vi "Scan and Trace(Normal Draft).vi"() -> ()   [LabVIEW 2020]
uses:
  <vilib>/Utility/error.llb/DialogType.ctl
  Global Parameters.vi
  <vilib>/DAQmx/miscellaneous.llb/DAQmx Fill In Error Info.vi
  <vilib>/DAQmx/configure/timing.llb/DAQmx Timing (Sample Clock).vi
  <vilib>/DAQmx/read.llb/DAQmx Read (Counter 1D U32 1Chan NSamp).vi
  <vilib>/DAQmx/create/channels.llb/DAQmx Create Channel (CI-Count Edges).vi
  <vilib>/Utility/file.llb/Write Delimited Spreadsheet (DBL).vi
  <resource>/objmgr/daqmx.rc
panel:
  out "Read + Move Time":u32=103
  out "Laser On":bool
  out "Current Position":dbl[](array[numeric])=[100.0, 99.99645996, 110.0]
  in  "stop":bool
  in  "Tab Control":T1(tab)
  in  "Graph path":path=path "I:/scan map test"
  out "Intensity Graph":dbl[][](graph)=[[95300.0, 98850.0, 103700.0, 104550.0, 102500.0, 51500.0, 51850.0, 19000.0, 20650.0, 15000.0, 15300.0, 17150.0, 16250.0, 17200.0, 14950.0, 15050.0, 17650.0, 15350.0, 14300.0, 14550.0, 15700.0], [77600.0, 97750.0, 99400.0, 99250.0, 95500.0, 53250.0, 25650.0, 18800.0, 17350.0, 14250.0, 17250.0, 16050.0, 15600.0, 15200.0, 15250.0, 15700.0, 15150.0, 14650.0, 15600.0, 15700.0, 16550.0], [97000.0, 96100.0, 101550.0, 99100.0, 97250.0, 50150.0, 23650.0, 21050.0, 17550.0, 15950.0, 15300.0, 14700.0, 15200.0, 16950.0, 14500.0, 15450.0, 14550.0, 17050.0, 14550.0, 14900.0, 16600.0], [95600.0, 95800.0, 102500.0, 99350.0, 94900.0, 52700.0, 26600.0, 21250.0, 16250.0, 16150.0, 14800.0, 15550.0, 15800.0, 16350.0, 15400.0, 15850.0, 14500.0, 14750.0, 15550.0, 15750.0, 14900.0], [100050.0, 96100.0, 94400.0, 100500.0, 94450.0, 54350.0, 23850.0, 18950.0, 16100.0, 14850.0, 16700.0, 14950.0, 14250.0, 16700.0, 16100.0, 15700.0, 16450.0, 14650.0, 16950.0, 14000.0, 15800.0], [100300.0, 96050.0, 96850.0, 98000.0, 90700.0, 51250.0, 23450.0, 18050.0, 18300.0, 17300.0, 17050.0, 16300.0, 15950.0, 14850.0, 15500.0, 16450.0, 16200.0, 17200.0, 16450.0, 15300.0, 17100.0], [95650.0, 95650.0, 100700.0, 98700.0, 94500.0, 53950.0, 25250.0, 18850.0, 17150.0, 16050.0, 15050.0, 15450.0, 16050.0, 14600.0, 16500.0, 16350.0, 15500.0, 15450.0, 15300.0, 15150.0, 15650.0], [96700.0, 96200.0, 96650.0, 103650.0, 93400.0, 53300.0, 22500.0, 19050.0, 15850.0, 15350.0, 16550.0, 15200.0, 15250.0, 15400.0, 16550.0, 13950.0, 15150.0, 15600.0, 15150.0, 14500.0, 15900.0], [97500.0, 98050.0, 101500.0, 101650.0, 97000.0, 53700.0, 23400.0, 19450.0, 16700.0, 16850.0, 16450.0, 16250.0, 15900.0, 14600.0, 15700.0, 15400.0, 14900.0, 15950.0, 15450.0, 16050.0, 16100.0], [95400.0, 97550.0, 102050.0, 98600.0, 92100.0, 61200.0, 24550.0, 20500.0, 16000.0, 15350.0, 14450.0, 14150.0, 15750.0, 15950.0, 15750.0, 14800.0, 15000.0, 16150.0, 17250.0, 15350.0, 17400.0], [95750.0, 92950.0, 96100.0, 96550.0, 92550.0, 90100.0, 21900.0, 23000.0, 15000.0, 15550.0, 16000.0, 16000.0, 15400.0, 14150.0, 14350.0, 15950.0, 17250.0, 15750.0, 16100.0, 15300.0, 14400.0]]
  in  "go to crusor":bool caption="X"
  in  "vertical num":u32=20
  in  "horizontal num":u32=10
  out "horizontal range":dbl=50.0
  in  "horizontal start":dbl=50.0
  out "vertical range":dbl=200.0
  in  "vertical start":dbl
  in  "Horizontal axis":i8(ring) items=["x", "y", "z", ""]
  in  "Vertical axis":i8(ring)=2 items=["x", "y", "z", ""]
  out "vertical step":dbl=10.0
  out "horizontal step":dbl=5.0
  in  "Stop scan":bool
  out "counts/s":dbl=14400.0 format="%#.10g"
  out "H goal position":dbl[](array[numeric])=[50.0, 55.0, 60.0, 65.0, 70.0, 75.0, 80.0, 85.0, 90.0, 95.0, 100.0]
  out "V goal position":dbl[](array[numeric])=[0.0, 10.0, 20.0, 30.0, 40.0, 50.0, 60.0, 70.0, 80.0, 90.0, 100.0, 110.0, 120.0, 130.0, 140.0, 150.0, 160.0, 170.0, 180.0, 190.0, 200.0]
  out "Loop  indicator":i32=2147483647
  in  "horizontal end":dbl=50.0
  in  "vertical end":dbl=200.0
  out "Waveform Chart":dbl(graph)=93500.0
  in  "Start moving":bool=TRUE
  in  "Save trace data?":bool
  in  "-0.05 2":bool caption="X"
  in  "Tracing axis":enum16{"x", "y", "z"}(ring)=enum."z"
  in  "-01 2":bool caption="X"
  in  "Wait time(ms)":u32
  in  "+01 2":bool caption="X"
  in  "+0.05 2":bool caption="X"
  in  "-0.01 2":bool caption="X"
  in  "+0.01 2":bool caption="X"
  in  "Exit Tracing":bool
  out "counts rate":dbl=93500.0 format="%#.10g"
  in  "Trace data file path 2":path=path "trace data"
  in  "set trace data save rate(ms)":u32
  in  "Stop Counts":bool
  out "Actual Duty Cycle":dbl=0.5
  out "Actual Frequency":dbl=50.0
  out "Duty Cycle":dbl=0.5 format="%.6f"
  out "Frequency":dbl=50.0 format="%.6f"
  out "Output Terminal":tag="/Dev1/PFI2"
  out "Counter":tag="Dev1/ctr0"
  out "Clock on":bool
  out "ASG连接状态":bool
  out "ASG error":errorcluster
  out "Scanner\n error":errorcluster
  out "Sample Clock Source":tag="/Dev1/PFI2"
  out "Sample Rate":dbl=50.0
  in  "Counter 2":tag="Dev1/ctr1"
  in  "Input Terminal":tag="/Dev1/PFI12"
  in  "Samples":i32=2
  out "Data":u32[](array[numeric])=[293, 581]
  in  "Active Edge":i32(ring)=10280 items=["Rising"=10280, "Falling"=10171]
  in  "Sample Mode":i32(ring)=10178 items=["Finite Samples"=10178, "Continuous Samples"=10123, "Hardware Timed Single Point"=12522]
  in  "milliseconds to wait":u32
  out "Position After move":dbl[](array[numeric]) format="%.6f"
  out "Position After move 2":dbl[](array[numeric]) format="%.6f"
  in  "start":bool
  in  "Select Process Before Start":enum16{"Goto cursor", "Trace", "Scan"}(ring)=enum."Trace"
  out "Scanning":bool
  out "Tracing":bool
  out "Goto cursor":bool
  # "Only for showing Clock Settings, Please go to Global Parameter to Change the Settings"
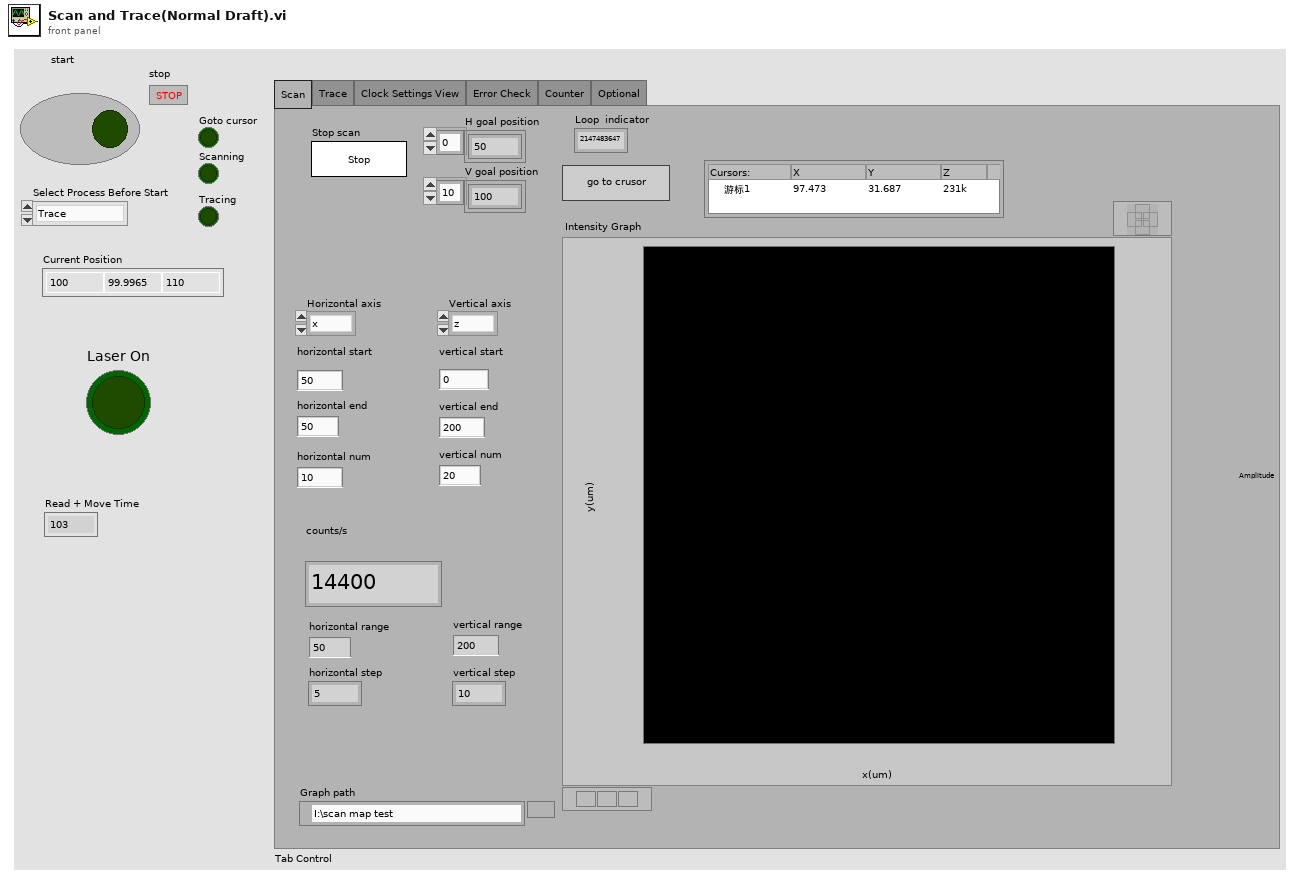
[diagram p1: front panel]
types:
  T1 = enum32{"Scan", "Trace", "Clock Settings View", "Error Check", "Counter", "Optional"}
  T2 = typedef "DialogType.ctl" = u16
  T3 = typedef "imagedata.ctl" = cluster{"image type":i32, "image depth":i32, "image":u8[], "mask":u8[], "colors":u32[], "Rectangle":cluster{"left":i16, "top":i16, "right":i16, "bottom":i16}}
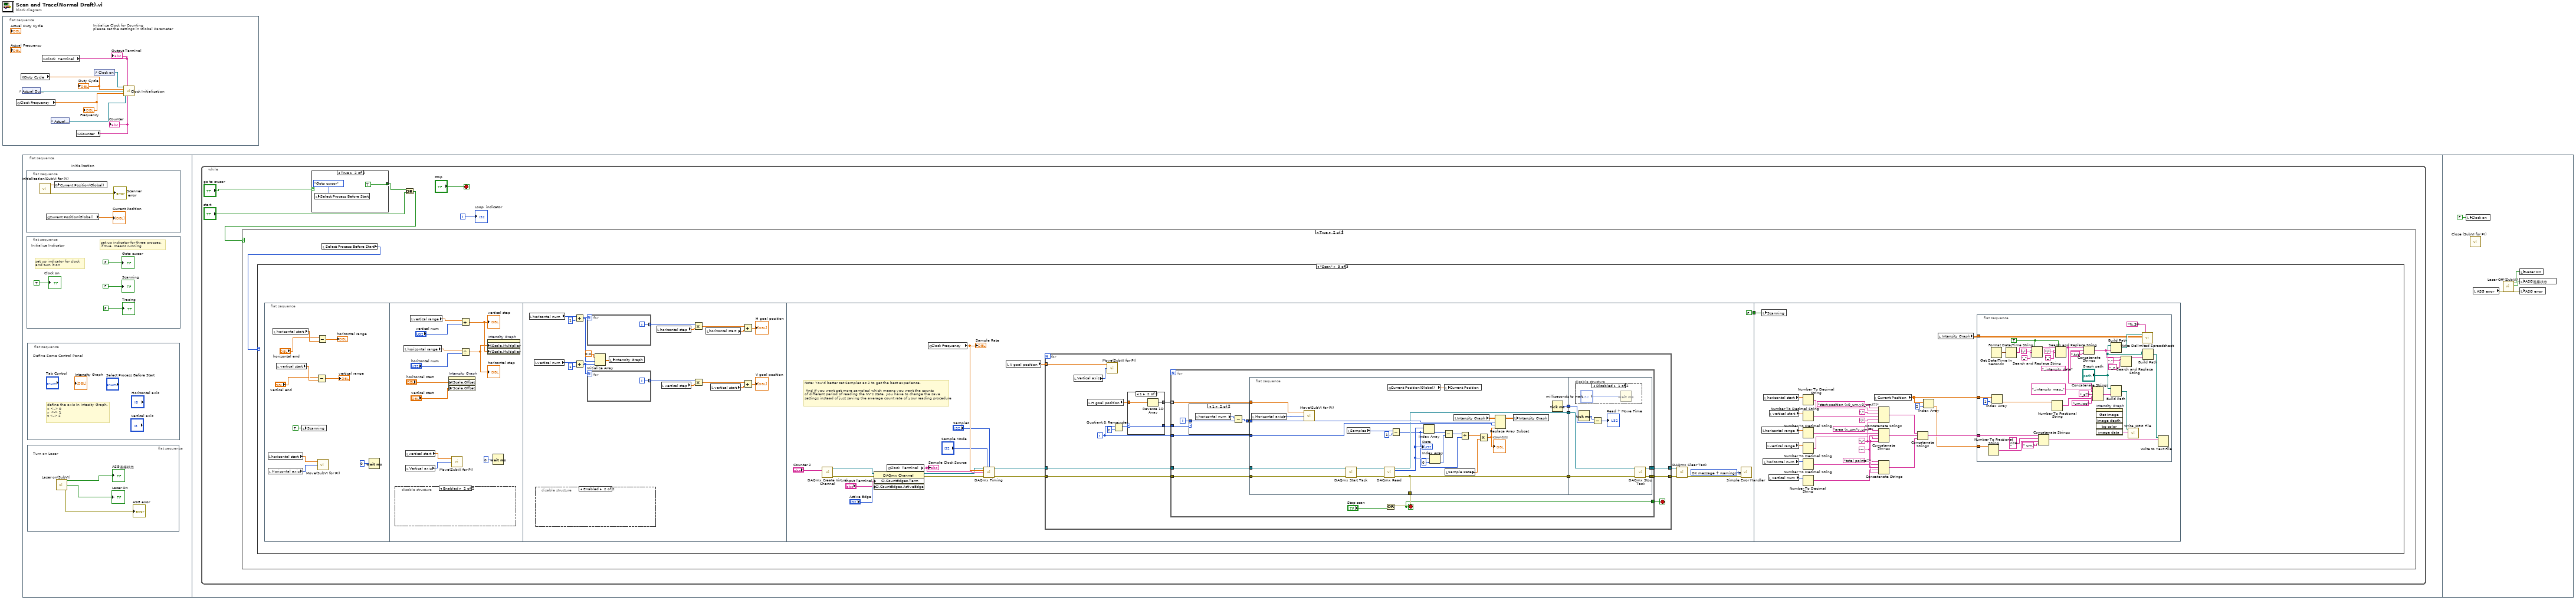
[diagram p0: block diagram]
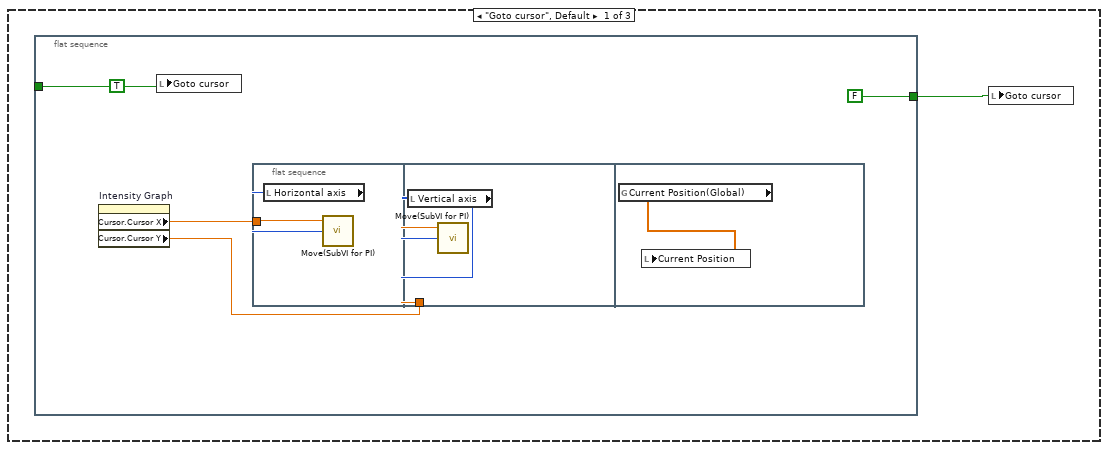
[diagram p3: hidden frame]
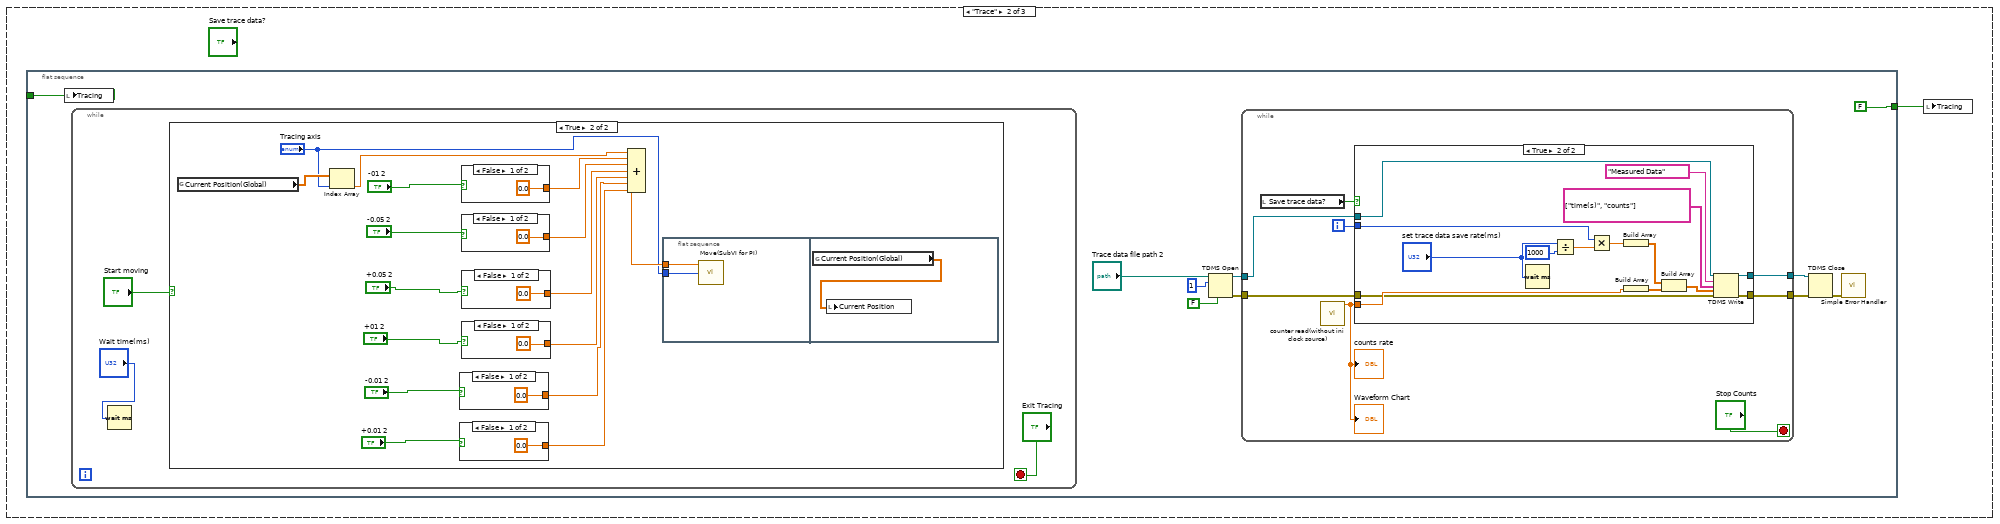
[diagram p4: hidden frame]
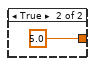
[diagram p7: hidden frame]
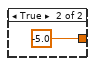
[diagram p8: hidden frame]
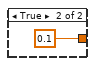
[diagram p9: hidden frame]
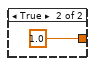
[diagram p10: hidden frame]
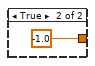
[diagram p11: hidden frame]
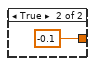
[diagram p12: hidden frame]
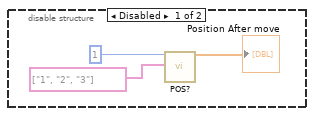
[diagram p13: hidden frame]
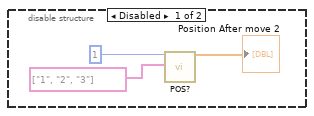
[diagram p14: hidden frame]
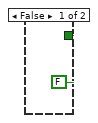
[diagram p18: hidden frame]
diagram:
  n1 = flat-sequence {
    frame #0 {
      # "Initialize Clock for Counting\nplease set the settings in Global Parameter"
      n2 = global read "Global Parameters.vi" "Clock Frequency"() -> (w3:dbl)
      "Frequency" <- w3
      n3 = global read "Global Parameters.vi" "Duty Cycle"() -> (w4:dbl)
      "Duty Cycle" <- w4
      n4 = control-ref of="Actual Duty Cycle"() -> (w1:refnum<vi>)
      n5 = global read "Global Parameters.vi" "Clock  Terminal"() -> (w5:tag)
      "Output Terminal" <- w5
      n6 = control-ref of="Actual Frequency"() -> (w2:refnum<vi>)
      n7 = global read "Global Parameters.vi" "Counter"() -> (w6:tag)
      "Counter" <- w6
      n8 = control-ref of="Clock on"() -> (w7:refnum<vi>)
      n9 = call "Clock Initialization.vi"("Boolean in"=w7, "Output Terminal"=w5, "Duty Cycle"=w4, "Actual Duty Cycle"=w1, "Frequency"=w3, "Actual Frequency"=w2, "Counter"=w6) -> ()  [unwired: 9 in]
    }
  }
  n10 = flat-sequence {
    frame #0 {
      # "Initialization"
      n11 = flat-sequence {
        frame #0 {
          n12 = call "Initialization(SubVI for PI).vi"() -> ("error out"=→"Scanner\n error":errorcluster, "Position"=w16:dbl[])  [unwired: 10 in]
          n13 = global read "Global Parameters.vi" "Current Position(Global)"() -> (→"Current Position":dbl[])
          n14 = global write "Global Parameters.vi" "Current Position(Global)"(w16) -> ()
        }
      }
      n15 = flat-sequence {
        frame #0 {
          # "Initialize Indicator"
          # "set up indicator for clock \nand turn it on"
          # "set up indicator for three prosses,\nif true, means running"
          "Goto cursor" <- FALSE
          "Tracing" <- FALSE
          "Scanning" <- FALSE
          "Clock on" <- TRUE
        }
      }
      n16 = flat-sequence {
        frame #0 {
          # "Define Some Control Panel"
          # "define the axis in Intesity Graph,\nx <-> 0\ny <-> 1\nz <-> 2"
        }
      }
      n17 = flat-sequence {
        frame #0 {
          # "Turn on Laser"
          n18 = call "Laser on(SubVI).vi"() -> ("error out"=→"ASG error":errorcluster, "Laser On"=→"Laser On":bool, "ASG Connection On?"=→"ASG连接状态":bool)  [unwired: 9 in]
        }
      }
    }
    frame #1 {
      n19 = while {
        i -> [w21]
        stop <- "stop" stop-if-true
        n20 = case shown="True" "go to crusor" {
          tunnel: [FALSE TRUE] -> w19
          frame False {
          }
          frame True {
            n21 = local write "Select Process Before Start"(enum16{"Goto cursor", "Trace", "Scan"}."Goto cursor" ("Select Process Before Start")) -> ()
          }
        }
        n22 = Or(x=w19, y="start") -> (x .or. y?=w18:bool)
        n23 = case shown="True" w18 {
          frame False {
          }
          frame True {
            n24 = local read "Select Process Before Start"() -> (w24:enum16{"Goto cursor", "Trace", "Scan"})
            n25 = case shown="\"Scan\"" w24 {
              frame "Goto cursor", Default {
                n26 = flat-sequence {
                  tunnel: TRUE -> [w28]
                  tunnel: [FALSE] -> w25
                  frame #0 {
                    n27 = property on="Intensity Graph" class="IntGraph (strict)"() -> ("Cursor.Cursor X"=w30:dbl, "Cursor.Cursor Y"=w29:dbl)  [unwired: 2 in, 2 out]
                    n28 = local write "Goto cursor"(w28) -> ()
                    n29 = flat-sequence {
                      tunnel: w30 -> [w32]
                      tunnel: w29 -> [w34]
                      frame #0 {
                        n30 = local read "Horizontal axis"() -> (w31:i8)
                        n31 = call "Move(SubVI for PI).vi"("Goal"=w32, "index"=w31) -> ()  [unwired: 5 in, 1 out]
                      }
                      frame #1 {
                        n32 = local read "Vertical axis"() -> (w33:i8)
                        n33 = call "Move(SubVI for PI).vi"("Goal"=w34, "index"=w33) -> ()  [unwired: 5 in, 1 out]
                      }
                      frame #2 {
                        n34 = global read "Global Parameters.vi" "Current Position(Global)"() -> (w35:dbl[])
                        n35 = local write "Current Position"(w35) -> ()
                      }
                    }
                  }
                }
                n36 = local write "Goto cursor"(w25) -> ()
              }
              frame "Trace" {
                n37 = flat-sequence {
                  tunnel: [FALSE] -> w37
                  tunnel: TRUE -> [w38]
                  frame #0 {
                    n38 = local write "Tracing"(w38) -> ()
                    n39 = while {
                      stop <- "Exit Tracing" stop-if-true
                      n40 = Wait (ms)(milliseconds to wait="Wait time(ms)") -> ()  [unwired: 1 out]
                      n41 = case shown="True" "Start moving" {
                        frame False {
                        }
                        frame True {
                          n42 = global read "Global Parameters.vi" "Current Position(Global)"() -> (w91:dbl[])
                          n43 = Index Array(array=w91, index="Tracing axis") -> (element=w84:dbl)
                          n44 = case shown="False" "-0.01 2" {
                            tunnel: [0.0 -5.0] -> w86
                            frame False {
                            }
                            frame True {
                            }
                          }
                          n45 = case shown="False" "+0.01 2" {
                            tunnel: [0.0 5.0] -> w85
                            frame False {
                            }
                            frame True {
                            }
                          }
                          n46 = case shown="False" "-01 2" {
                            tunnel: [0.0 -0.1] -> w90
                            frame False {
                            }
                            frame True {
                            }
                          }
                          n47 = case shown="False" "-0.05 2" {
                            tunnel: [0.0 -1.0] -> w89
                            frame False {
                            }
                            frame True {
                            }
                          }
                          n48 = case shown="False" "+0.05 2" {
                            tunnel: [0.0 1.0] -> w88
                            frame False {
                            }
                            frame True {
                            }
                          }
                          n49 = case shown="False" "+01 2" {
                            tunnel: [0.0 0.1] -> w87
                            frame False {
                            }
                            frame True {
                            }
                          }
                          n50 = Compound Arithmetic op=ADD(w84, w90, w89, w88, w87, w86, w85) -> (w77:dbl)
                          n51 = flat-sequence {
                            tunnel: w77 -> [w105]
                            tunnel: "Tracing axis" -> [w104]
                            frame #0 {
                              n52 = call "Move(SubVI for PI).vi"("Goal"=w105, "index"=w104) -> ()  [unwired: 5 in, 1 out]
                            }
                            frame #1 {
                              n53 = global read "Global Parameters.vi" "Current Position(Global)"() -> (w106:dbl[])
                              n54 = local write "Current Position"(w106) -> ()
                            }
                          }
                        }
                      }
                    }
                    n55 = TDMS Open(6:FALSE ("disable buffering (T)"), 10:1, 11:"Trace data file path 2") -> (0:w45:errorcluster, 3:w44:refnum<k34>)  [unwired: 4 in]
                    n56 = while {
                      tunnel: w45 -> [w54]
                      tunnel: w44 -> [w53]
                      tunnel: [w50] -> w42
                      tunnel: [w49] -> w41
                      i -> [w55]
                      stop <- "Stop Counts" stop-if-true
                      n57 = local read "Save trace data?"() -> (w51:bool)
                      n58 = call "counter read(without ini clock source).vi"() -> ("counter rate"=w52:dbl)  [unwired: 11 in]
                      "counts rate" <- w52
                      "Waveform Chart" <- w52
                      n59 = case shown="True" w51 {
                        tunnel: w53 -> [w57 w64]
                        tunnel: [w57 w63] -> w50
                        tunnel: w52 -> [_ w62]
                        tunnel: w54 -> [w56 w61]
                        tunnel: [w56 w60] -> w49
                        tunnel: w55 -> [_ w59]
                        frame False {
                        }
                        frame True {
                          n60 = Wait (ms)(milliseconds to wait="set trace data save rate(ms)") -> ()  [unwired: 1 out]
                          n61 = Divide(x="set trace data save rate(ms)", y=u32 1000) -> (x/y=w66:dbl)
                          n62 = Multiply(x=w59, y=w66) -> (x*y=w65:dbl)
                          n63 = Build Array(w65) -> (w70:dbl[])
                          n64 = Build Array(w62) -> (w69:dbl[])
                          n65 = Build Array(w70, w69) -> (w68:dbl[][])
                          n66 = TDMS Write(0:w64, 5:"Measured Data" ("group name"), 7:string[] ["time(s)", "counts"] ("channel names"), 9:w68, 11:w61) -> (4:w63:refnum<k34>, 15:w60:errorcluster)  [unwired: 1 in, 2 out]
                        }
                      }
                    }
                    n67 = TDMS Close(8:w41, 11:w42) -> (0:w43:errorcluster)  [unwired: 1 out]
                    n68 = call <vilib>:"Simple Error Handler.vi"("error in (no error)"=w43) -> ()  [unwired: 1 in, 8 out]
                  }
                }
                n69 = local write "Tracing"(w37) -> ()
              }
              frame "Scan" {
                n70 = flat-sequence {
                  tunnel: [FALSE] -> w107
                  tunnel: w107 -> [w271]
                  frame #0 {
                    n71 = local read "horizontal start"() -> (w109:dbl)
                    n72 = local read "Horizontal axis"() -> (w110:i8)
                    n73 = local read "horizontal start"() -> (w114:dbl)
                    n74 = local read "vertical start"() -> (w112:dbl)
                    n75 = local write "Scanning"(TRUE) -> ()
                    n76 = Subtract(x="vertical end", y=w112) -> (x-y=→"vertical range":dbl)
                    n77 = Subtract(x="horizontal end", y=w114) -> (x-y=→"horizontal range":dbl)
                    n78 = call "Move(SubVI for PI).vi"("Goal"=w109, "index"=w110) -> ()  [unwired: 5 in, 1 out]
                    n79 = Wait (ms)(milliseconds to wait=u32 0 ("milliseconds to wait 2")) -> ()  [unwired: 1 out]
                  }
                  frame #1 {
                    n80 = disable-structure shown="Enabled" {
                      frame Disabled {
                        n81 = call "POS?.vi"("System no."=1, "Axes to query"=string[] ["1", "2", "3"] ("String")) -> ("Position"=→"Position After move":dbl[])  [unwired: 3 in, 14 out]
                      }
                      frame Enabled {
                      }
                    }
                    n82 = local read "horizontal range"() -> (w122:dbl)
                    n83 = local read "vertical start"() -> (w119:dbl)
                    n84 = local read "Vertical axis"() -> (w120:i8)
                    n85 = local read "vertical range"() -> (w121:dbl)
                    n86 = property on="Intensity Graph" class="IntGraph (strict)"("XScale.Offset"="horizontal start", "YScale.Offset"="vertical start") -> ()  [unwired: 2 in, 2 out]
                    n87 = call "Move(SubVI for PI).vi"("Goal"=w119, "index"=w120) -> ()  [unwired: 5 in, 1 out]
                    n88 = Divide(x=w121, y="vertical num") -> (x/y=w123:dbl)
                    "vertical step" <- w123
                    n89 = Divide(x=w122, y="horizontal num") -> (x/y=w124:dbl)
                    "horizontal step" <- w124
                    n90 = property on="Intensity Graph" class="IntGraph (strict)"("XScale.Multiplier"=w124, "YScale.Multiplier"=w123) -> ()  [unwired: 2 in, 2 out]
                    n91 = Wait (ms)(milliseconds to wait=u32 0 ("milliseconds to wait 2")) -> ()  [unwired: 1 out]
                  }
                  frame #2 {
                    n92 = local read "horizontal num"() -> (w134:u32)
                    n93 = local read "vertical num"() -> (w137:u32)
                    n94 = disable-structure shown="Enabled" {
                      frame Disabled {
                        n95 = call "POS?.vi"("System no."=1, "Axes to query"=string[] ["1", "2", "3"] ("String")) -> ("Position"=→"Position After move 2":dbl[])  [unwired: 3 in, 14 out]
                      }
                      frame Enabled {
                      }
                    }
                    n96 = Add(x=w134, y=1) -> (x+y=w133:u32)
                    n97 = Add(x=w137, y=1) -> (x+y=w132:u32)
                    n98 = for {
                      N: w133 -> [_]
                      tunnel: [w154] -> w149 mode=indexing
                      i -> [w154]
                    }
                    n99 = for {
                      N: w132 -> [_]
                      tunnel: [w153] -> w144 mode=indexing
                      i -> [w153]
                    }
                    n100 = Initialize Array(0.0, w133, w132) -> (w138:dbl[][])
                    n101 = local write "Intensity Graph"(w138) -> ()
                    n102 = local read "horizontal step"() -> (w148:dbl)
                    n103 = local read "vertical step"() -> (w143:dbl)
                    n104 = Multiply(x=w149, y=w148) -> (x*y=w147:dbl[])
                    n105 = Multiply(x=w144, y=w143) -> (x*y=w142:dbl[])
                    n106 = local read "horizontal start"() -> (w146:dbl)
                    n107 = local read "vertical start"() -> (w141:dbl)
                    n108 = Add(x=w147, y=w146) -> (x+y=→"H goal position":dbl[])
                    n109 = Add(x=w142, y=w141) -> (x+y=→"V goal position":dbl[])
                  }
                  frame #3 {
                    w170 = T2 3 items=["no dialog", "OK message", "continue or stop message", "OK message + warnings", "continue/stop + warnings"] ("type of dialog (OK msg:1)")
                    # "Note: You'd better set Samples as 2 to get the best experience,\n\n And if you want get more samples( which means you want the counts \nof different period of reading the NV's state, you have to change the save \nsettings instead of just saving the average count rate of your reading procedure"
                    n110 = call-poly <vilib>:"DAQmx Create Virtual Channel.vi"("counter"="Counter 2") -> ("task out"=w166:refnum<k21>, "error out"=w165:errorcluster)  [unwired: 13 in]
                    n111 = property class="DAQmx Channel"(reference=w166, error in=w165, "CI.CountEdges.Term"="Input Terminal", "CI.CountEdges.ActiveEdge"="Active Edge") -> (reference out=w158:refnum<k21>, error out=w157:errorcluster)
                    n112 = global read "Global Parameters.vi" "Clock  Terminal"() -> (w163:tag)
                    "Sample Clock Source" <- w163
                    n113 = global read "Global Parameters.vi" "Clock Frequency"() -> (w164:dbl)
                    "Sample Rate" <- w164
                    n114 = call-poly <vilib>:"DAQmx Timing.vi"("task/channels in"=w158, "sample mode"="Sample Mode", "samples per channel"="Samples", "rate"=w164, "source"=w163, "error in"=w157) -> ("task out"=w156:refnum<k21>, "error out"=w155:errorcluster)  [unwired: 8 in]
                    n115 = local read "V goal position"() -> (w173:dbl[])
                    n116 = for {
                      tunnel: w173 -> [w180] mode=indexing
                      tunnel: [w175] -> w162
                      tunnel: [w174] -> w161
                      tunnel: w156 -> [w177]
                      tunnel: w155 -> [w176]
                      i -> [w181]
                      stop <- w178 stop-if-true
                      n117 = local read "Vertical axis"() -> (w179:i8)
                      n118 = local read "H goal position"() -> (w185:dbl[])
                      n119 = call "Move(SubVI for PI).vi"("Goal"=w180, "index"=w179) -> ()  [unwired: 5 in, 1 out]
                      n120 = Quotient & Remainder(x=w181, y=2) -> (x-y*floor(x/y)=w184:i32)  [unwired: 1 out]
                      n121 = case shown="1" w184 {
                        selector: w184 -> [w239 w241]
                        tunnel: w185 -> [w240 w243]
                        tunnel: [w240 w242] -> w183
                        tunnel: [w239 w241] -> w182
                        frame 0, Default {
                        }
                        frame 1 {
                          n122 = Reverse 1D Array(array=w243) -> (reversed array=w242:dbl[])
                        }
                      }
                      n123 = for {
                        tunnel: w183 -> [w201] mode=indexing
                        tunnel: w182 -> [w200]
                        tunnel: w181 -> [w197]
                        tunnel: [w194] -> w178
                        tunnel: w177 -> [w193]
                        tunnel: w176 -> [w192]
                        tunnel: [w189] -> w175
                        tunnel: [w188] -> w174
                        i -> [w199]
                        stop <- w194 stop-if-true
                        n124 = case shown="1" w200 {
                          tunnel: w199 -> [w202 w204]
                          tunnel: [w202 w203] -> w198
                          frame 0, Default {
                          }
                          frame 1 {
                            n125 = local read "horizontal num"() -> (w205:u32)
                            n126 = Subtract(x=w205, y=w204) -> (x-y=w203:u32)
                          }
                        }
                        n127 = flat-sequence {
                          tunnel: [w221] -> w196
                          tunnel: [w222] -> w191
                          tunnel: [w221] -> w190
                          tunnel: [w208] -> w187
                          tunnel: w198 -> [w229]
                          tunnel: w201 -> [w207]
                          tunnel: w197 -> [w228]
                          tunnel: w193 -> [w224]
                          tunnel: w192 -> [w223]
                          tunnel: w191 -> [w236]
                          tunnel: w190 -> [w235]
                          tunnel: [w234] -> w189
                          tunnel: [w233] -> w188
                          tunnel: w187 -> [w232]
                          frame #0 {
                            n128 = local read "Horizontal axis"() -> (w206:i8)
                            n129 = call "Move(SubVI for PI).vi"("Goal"=w207, "index"=w206) -> ()  [unwired: 5 in, 1 out]
                            n130 = call <vilib>:"DAQmx Start Task.vi"("task/channels in"=w224, "error in"=w223) -> ("task out"=w210:refnum<k21>, "error out"=w209:errorcluster)  [unwired: 12 in]
                            n131 = local read "Samples"() -> (w215:i32)
                            n132 = call-poly <vilib>:"DAQmx Read.vi"("task/channels in"=w210, "error in"=w209) -> ("task out"=w222:refnum<k21>, "data"=w214:u32[], "error out"=w221:errorcluster)  [unwired: 11 in]
                            "Data" <- w214
                            n133 = global read "Global Parameters.vi" "Current Position(Global)"() -> (w226:dbl[])
                            n134 = Subtract(x=w215, y=1) -> (x-y=w211:i32)
                            n135 = Index Array(array=w214, index=w211) -> (element=w217:u32)
                            n136 = Index Array(array=w214, index=0) -> (element=w218:u32)
                            n137 = Subtract(x=w217, y=w218) -> (x-y=w216:u32)
                            n138 = local write "Current Position"(w226) -> ()
                            n139 = local read "Sample Rate"() -> (w212:dbl)
                            n140 = local read "Intensity Graph"() -> (w230:dbl[][])
                            n141 = Divide(x=w216, y=w211) -> (x/y=w213:dbl)
                            n142 = Multiply(x=w213, y=w212) -> (x*y=w225:dbl)
                            "counts/s" <- w225
                            n143 = Replace Array Subset(array=w230, new element=w225, index (row)=w229, index (col)=w228) -> (w227:dbl[][])
                            n144 = local write "Intensity Graph"(w227) -> ()
                            n145 = Tick Count (ms)() -> (millisecond timer value=w208:u32)
                          }
                          frame #1 {
                            n146 = disable-structure shown="Disabled" {
                              frame Disabled {
                                n147 = Wait (ms)(milliseconds to wait="milliseconds to wait") -> ()  [unwired: 1 out]
                              }
                              frame Enabled {
                              }
                            }
                            n148 = Tick Count (ms)() -> (millisecond timer value=w231:u32)
                            n149 = Subtract(x=w231, y=w232) -> (x-y=→"Read + Move Time":u32)
                            n150 = call <vilib>:"DAQmx Stop Task.vi"("task/channels in"=w236, "error in"=w235) -> ("task out"=w234:refnum<k21>, "error out"=w233:errorcluster)  [unwired: 12 in]
                          }
                        }
                        n151 = Or(x=w196, y="Stop scan") -> (x .or. y?=w194:bool)
                      }
                    }
                    n152 = call <vilib>:"DAQmx Clear Task.vi"("task in"=w162, "error in"=w161) -> ("error out"=w171:errorcluster)  [unwired: 13 in]
                    n153 = call <vilib>:"Simple Error Handler.vi"("type of dialog (OK msg:1)"=w170, "error in (no error)"=w171) -> ()  [unwired: 3 in, 5 out]
                  }
                  frame #4 {
                    w260 = "\r"
                    w262 = "*" ("string")
                    n154 = local write "Scanning"(w271) -> ()
                    n155 = local read "horizontal range"() -> (w249:dbl)
                    n156 = local read "horizontal num"() -> (w255:u32)
                    n157 = local read "horizontal start"() -> (w252:dbl)
                    n158 = local read "vertical range"() -> (w248:dbl)
                    n159 = local read "vertical num"() -> (w254:u32)
                    n160 = local read "vertical start"() -> (w251:dbl)
                    n161 = Number To Decimal String(number=w252) -> (decimal integer string=w269:string)  [unwired: 1 out]
                    n162 = Number To Decimal String(number=w251) -> (decimal integer string=w267:string)  [unwired: 1 out]
                    n163 = Number To Decimal String(number=w249) -> (decimal integer string=w264:string)  [unwired: 1 out]
                    n164 = Number To Decimal String(number=w248) -> (decimal integer string=w250:string)  [unwired: 1 out]
                    n165 = Number To Decimal String(number=w255) -> (decimal integer string=w261:string)  [unwired: 1 out]
                    n166 = Number To Decimal String(number=w254) -> (decimal integer string=w253:string)  [unwired: 1 out]
                    n167 = local read "Current Position"() -> (w244:dbl[])
                    n168 = Concatenate Strings("start position (x0_um,y0_um)=(" ("string"), w269, "," ("string"), w267, ")" ("string"), w260) -> (w259:string)
                    n169 = Concatenate Strings("area (x_um*y_um)=" ("string"), w264, w262, w250, w260) -> (w258:string)
                    n170 = Concatenate Strings("total points=" ("string"), w261, w262, w253, w260) -> (w257:string)
                    n171 = Concatenate Strings(w259, w258, w257) -> (w256:string)
                    n172 = Index Array(array=w244, index=2) -> (element=w246:dbl)
                    n173 = local read "Intensity Graph"() -> (w245:dbl[][])
                    n174 = flat-sequence {
                      tunnel: w245 -> [w274]
                      tunnel: w256 -> [w287]
                      tunnel: w246 -> [w285]
                      tunnel: w244 -> [w280]
                      frame #0 {
                        w277 = TRUE ("replace all? (F)")
                        n175 = Number To Fractional String(number=w285) -> (F-format string=w284:string)  [unwired: 3 in]
                        n176 = Get Date/Time In Seconds() -> (seconds since 1Jan1904=w307:timestamp)
                        n177 = Index Array(array=w280, index=2 ("索引")) -> (element=w278:dbl)
                        n178 = Format Date/Time String(seconds (now)=w307) -> (date/time string=w301:string)  [unwired: 2 out]
                        n179 = Search and Replace String(replace all?=w277, input string=w301, search string=":", replace string="_" ("replace string (\"\")")) -> (result string=w304:string)  [unwired: 1 in, 6 out]
                        n180 = Concatenate Strings(w287, "\nz=" ("字符串"), w284, " um." ("字符串")) -> (w286:string)
                        n181 = Number To Fractional String(number=w278) -> (F-format string=w281:string)  [unwired: 3 in]
                        n182 = Search and Replace String(replace all?=w277, input string=w304, search string="/", replace string="_" ("replace string (\"\")")) -> (result string=w292:string)  [unwired: 1 in, 6 out]
                        n183 = Concatenate Strings(w292, "_intensity date" ("string"), ".txt" ("string")) -> (w297:string)
                        n184 = Concatenate Strings(w292, "_intensity map_" ("string"), "_z=" ("字符串"), w281, "um.jpg" ("string")) -> (w300:string)
                        n185 = invoke on="Intensity Graph" class="IntGraph (strict)" method="Get Image"() -> ("image data"=w273:T3)  [unwired: 6 in, 5 out]
                        n186 = Build Path(base path="Graph path", name or relative path=w297) -> (appended path=w275:path)
                        n187 = Build Path(base path="Graph path", name or relative path=w300) -> (appended path=w299:path)
                        n188 = Search and Replace String(input string=w297, search string="." ("substring (\"\")"), replace string="_2." ("replace string (\"\")")) -> (result string=w294:string)  [unwired: 1 in, 7 out]
                        n189 = call <vilib>:"Write JPEG File.vi"("image data"=w273, "path to JPEG file"=w299) -> ()  [unwired: 1 in, 9 out]
                        n190 = call-poly <vilib>:"Write Delimited Spreadsheet.vi"("file path (dialog if empty)"=w275, "format (%.3f)"="%.3f", "2D data"=w274) -> ()  [unwired: 11 in, 2 out]
                        n191 = Build Path(base path="Graph path", name or relative path=w294) -> (appended path=w293:path)
                        n192 = Write to Text File(file (use dialog)=w293, text=w286) -> ()  [unwired: 1 in, 4 out]
                      }
                    }
                  }
                }
              }
            }
          }
        }
        "Loop  indicator" <- w21
      }
    }
    frame #2 {
      n193 = local write "Clock on"(FALSE) -> ()
      n194 = call "Close (SubVI for PI).vi"() -> ()  [unwired: 12 in]
      n195 = local read "ASG error"() -> (w311:errorcluster)
      n196 = call "Laser Off (SubVI).vi"("error in (no error)"=w311) -> ("error out"=w312:errorcluster, "ASG Connection on"=w313:bool, "Laser On"=w314:bool)  [unwired: 8 in]
      n197 = local write "Laser On"(w314) -> ()
      n198 = local write "ASG连接状态"(w313) -> ()
      n199 = local write "ASG error"(w312) -> ()
    }
  }
